vi "VCS Set Position Marker Parameter.vi"(8 "error in (no error)":errorcluster, 9 "position marker parameter":T1 {"positionMarkerMode" items=["continuous", "single", "multiple"]; "positionMarkerEdgeType" items=["both edges", "rising edge", "falling edge"]}, 11 "axis in":cluster{"keyHandle":u32, "nodeId":u16}={"keyHandle"=0, "nodeId"=1}) -> (0 "error out":errorcluster, 3 "axis out":cluster{"keyHandle":u32, "nodeId":u16}={"keyHandle"=0, "nodeId"=1})   [LabVIEW 2019, in "maxonEPOS.lvlib"]
doc: "<B>VCS_SetPositionMarkerParameter</B> writes all parameters for position marker method."
uses:
  Examples/maxonEPOS.lvlib
  Resources/EposCmd.dll
  Resources/EposCmd64.dll
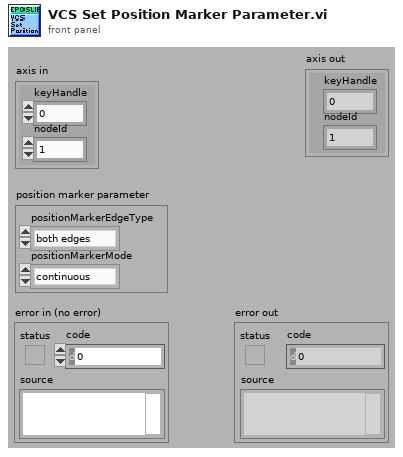
[diagram p1: front panel]
types:
  T1 = cluster{"positionMarkerEdgeType":u8, "positionMarkerMode":u8}
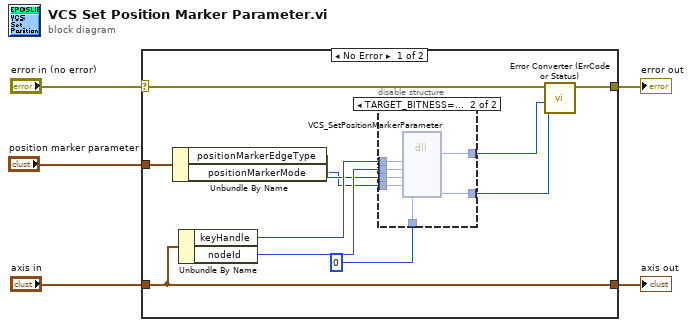
[diagram p0: block diagram]
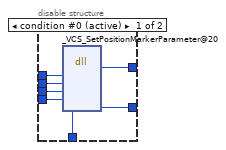
[diagram p2: hidden frame]
diagram:
  n1 = case shown="No Error" "error in (no error)" {
    selector: "error in (no error)" -> [w14 w31]
    tunnel: "axis in" -> [w16 w32]
    tunnel: [w16 w32] -> w4
    tunnel: [w15 w31] -> w3
    tunnel: "position marker parameter" -> [w8 _]
    frame No Error {
      n2 = Unbundle By Name(w8) -> ("positionMarkerEdgeType"=w7:u8, "positionMarkerMode"=w6:u8)
      n3 = Unbundle By Name(w16) -> ("keyHandle"=w13:u32, "nodeId"=w12:u16)
      n4 = disable-structure shown="TARGET_BITNESS==64" {
        disable-tunnel: w13 -> [w23 w30]
        disable-tunnel: w12 -> [w22 w29]
        disable-tunnel: u32 0 ("pErrorCode") -> [w21 w28]
        disable-tunnel: [w20 w27] -> w10
        disable-tunnel: [w19 w26] -> w9
        disable-tunnel: w7 -> [w18 w25]
        disable-tunnel: w6 -> [w17 w24]
        frame condition #0 (active) {
          n5 = dll-call lib="C:/workspace/project/scancon/sw/SSI_Tool/InstrumentsInterfaces/Motordriver/maxon EPOS/Resources/EposCmd.*" fn="_VCS_SetPositionMarkerParameter@20"("KeyHandle"=w23, "NodeId"=w22, "PositionMarkerEdgeType"=w18, "PositionMarkerMode"=w17, "pErrorCode"=w21) -> (w19:i32, "pErrorCode"=w20:u32)  [unwired: 7 in, 2 out]
        }
        frame condition #1 {
          n6 = dll-call lib="C:/setup/Resources/EposCmd64.*" fn="VCS_SetPositionMarkerParameter" ("EposCmd.dll:_VCS_SetPositionMarkerParameter@20")("KeyHandle"=w30, "NodeId"=w29, "PositionMarkerEdgeType"=w25, "PositionMarkerMode"=w24, "pErrorCode"=w28) -> ("Rückgabetyp"=w26:i32, "pErrorCode"=w27:u32)  [unwired: 7 in, 2 out]
        }
      }
      n7 = call "Error Converter (ErrCode or Status).vi"("error code"=w10, "return type"=w9, "error in (no error)"=w14) -> ("error out"=w15:errorcluster)  [unwired: 7 in]
    }
    frame Error {
    }
  }
  "error out" <- w3
  "axis out" <- w4
